vi "A33LoadArbitraryVolat.vi"(0 "VISA resource name":refnum<visa-resource-name>, 1 "ARB Number":u32=1, 3 "WFM Source":u16(ring) items=["Single file", "Split files", "Array"], 5 "Channel (1: Channel1)":u16(ring)=1 items=["Channel1"=1, "Channel2"=2], 6 "Array WFM":i16[](array[numeric]), 8 "WFM (Column) Number":i32, 9 "WFM Path":path, 11 "error in (no error)":errorcluster, 12 "WFM Length":i32, 14 "Timeout (40000 ms)":u32=40000) -> (4 "VISA resource name out":refnum<visa-resource-name>, 10 "Length of string written":i32, 15 "error out":errorcluster)   [LabVIEW 2022 SP3]
doc: "Creates and saves an arbitrary waveform in edit memory. \n\n<B>Note:</B>\n\nCreates an arbitrary waveform in edit memory and because of this, the waveform will remain stored on the instrument until deleted. If any sensitive information is contained in the arbitrary waveform, it is recommended that the waveform be deleted when finished."
uses:
  <vilib>/Utility/file.llb/Read From Spreadsheet File (I64).vi
panel:
  out "Attempts":i32
  # "Load waveform into arb\nmemory of a certain channel\nunder name 'ARB#'\nIf WFM alerady exists - use ClearArbitrary\n64M points in total per channel\nTimeout is not implemented, because this\nVI is inline-compatible, need external timeout\nincrease"
  # "No dots in the file name!"
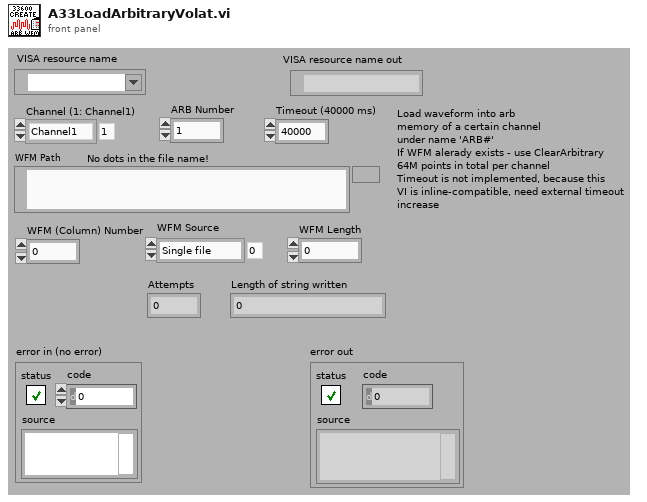
[diagram p1: front panel]
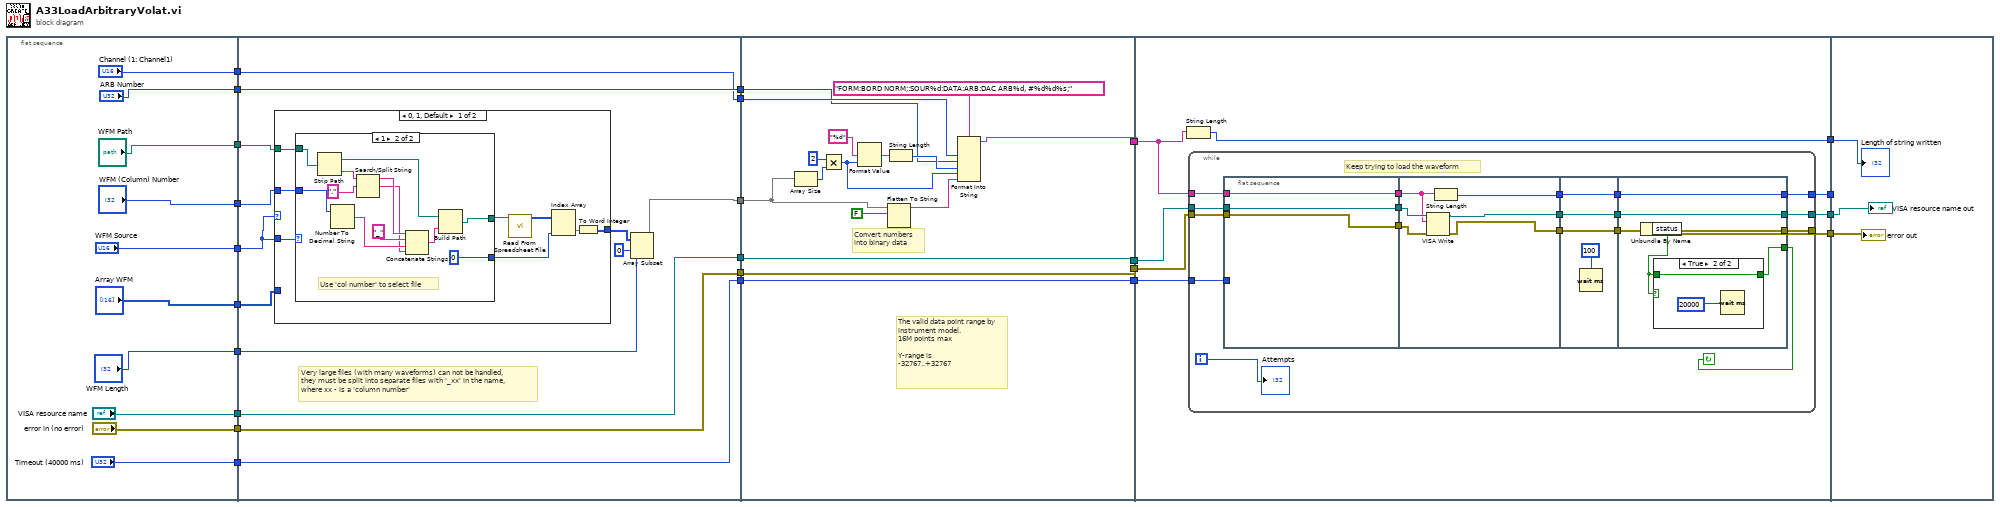
[diagram p0: block diagram]
diagram:
  n1 = flat-sequence {
    tunnel: ["Array WFM"] -> w12
    tunnel: ["WFM Source"] -> w11
    tunnel: ["ARB Number"] -> w10
    tunnel: ["Channel (1: Channel1)"] -> w9
    tunnel: ["error in (no error)"] -> w8
    tunnel: ["VISA resource name"] -> w7
    tunnel: ["Timeout (40000 ms)"] -> w6
    tunnel: ["WFM Length"] -> w5
    tunnel: ["WFM (Column) Number"] -> w4
    tunnel: ["WFM Path"] -> w3
    tunnel: [w38] -> w18
    tunnel: [w39] -> w17
    tunnel: [w40] -> w16
    tunnel: [w45] -> w15
    tunnel: [w41] -> w14
    tunnel: [w42] -> w13
    tunnel: w12 -> [w44]
    tunnel: w11 -> [w43]
    tunnel: w10 -> [w42]
    tunnel: w9 -> [w41]
    tunnel: w8 -> [w40]
    tunnel: w7 -> [w39]
    tunnel: w6 -> [w38]
    tunnel: w5 -> [w37]
    tunnel: w4 -> [w36]
    tunnel: w3 -> [w35]
    tunnel: [w86] -> w22
    tunnel: [w85] -> w21
    tunnel: [w84] -> w20
    tunnel: [w71] -> w19
    tunnel: w18 -> [w86]
    tunnel: w17 -> [w85]
    tunnel: w16 -> [w84]
    tunnel: w15 -> [w72]
    tunnel: w14 -> [w76]
    tunnel: w13 -> [w75]
    tunnel: [w91] -> w24
    tunnel: [w90] -> w23
    tunnel: w22 -> [w94]
    tunnel: w21 -> [w93]
    tunnel: w20 -> [w92]
    tunnel: w19 -> [w88]
    tunnel: [w89] -> w2
    tunnel: [w87] -> w1
    tunnel: w24 -> [w135]
    tunnel: w23 -> [w136]
    tunnel: w2 -> [_]
    tunnel: w1 -> [w134]
    frame #0 {
    }
    frame #1 {
      # "Very large files (with many waveforms) can not be handled,\nthey must be split into separate files with '_xx' in the name,\nwhere xx - is a 'column number'"
      n2 = case shown="0, 1, Default" w43 {
        tunnel: [w49 w70] -> w47
        tunnel: w35 -> [w54 _]
        tunnel: w36 -> [w53 _]
        tunnel: w43 -> [w50 _]
        tunnel: w44 -> [_ w70]
        frame 0, 1, Default {
          n3 = case shown="1" w50 {
            tunnel: w54 -> [w57 w69]
            tunnel: w53 -> [w56 w66]
            tunnel: [w57 w59] -> w52
            tunnel: [w56 0 ("x")] -> w51
            frame 0, Default {
              # "File contains multiple wfms"
            }
            frame 1 {
              # "Use 'col number' to select file"
              n4 = Strip Path(path=w69) -> (stripped path=w61:path, name=w67:string)
              n5 = Number To Decimal String(number=w66) -> (decimal integer string=w63:string)  [unwired: 1 in]
              n6 = Search/Split String(string=w67, search string/char (-)=".") -> (substring before match=w65:string, match + rest of string=w62:string)  [unwired: 1 in, 1 out]
              n7 = Concatenate Strings(w65, "_", w63, w62) -> (w60:string)
              n8 = Build Path(base path=w61, name or relative path=w60) -> (appended path=w59:path)
            }
          }
          n9 = call-poly <vilib>:"Read From Spreadsheet File.vi"("file path (dialog if empty)"=w52) -> ("all rows"=w55:i64[][])  [unwired: 6 in, 4 out]
          n10 = Index Array(array=w55, index (col)=w51) -> (element=w48:i64[])  [unwired: 1 in]
          n11 = To Word Integer(number=w48) -> (16bit integer=w49:i16[])
        }
        frame 2 {
        }
      }
      n12 = Array Subset(array=w47, index=0 ("x"), length=w37) -> (w45:i16[])
    }
    frame #2 {
      # "Convert numbers\ninto binary data"
      # "The valid data point range by instrument model. \n16M points max\n\nY-range is\n-32767..+32767"
      n13 = Array Size(array=w72) -> (size(s)=w79:i32)
      n14 = Multiply(x=2, y=w79) -> (x*y=w82:i32)
      n15 = Format Value(format string="%d", value (0)=w82) -> (output string=w80:string)  [unwired: 1 in]
      n16 = Flatten To String(anything=w72, prepend array or string size? (T)=FALSE) -> (data string=w83:string)  [unwired: 2 in, 2 out]
      n17 = String Length(string=w80) -> (length=w81:i32)
      n18 = Format Into String(format string="FORM:BORD NORM;:SOUR%d:DATA:ARB:DAC ARB%d, #%d%d%s;" ("string"), w76, w75, w81, w82, w83) -> (resulting string=w71:string)  [unwired: 2 in, 1 out]
    }
    frame #3 {
      n19 = String Length(string=w88) -> (length=w87:i32)
      n20 = while {
        tunnel: w88 -> [w109]
        tunnel: w94 -> [w108]
        tunnel: w93 -> [w107]
        tunnel: w92 -> [w106]
        tunnel: [w105] -> w91
        tunnel: [w104] -> w90
        tunnel: [w95] -> w89
        i -> [w98]
        stop <- w103 continue-if-true
        # "Keep trying to load the waveform"
        n21 = flat-sequence {
          tunnel: [w113] -> w112
          tunnel: [w114] -> w111
          tunnel: w109 -> [w115]
          tunnel: [w115] -> w110
          tunnel: w108 -> [_]
          tunnel: w107 -> [w113]
          tunnel: w106 -> [w114]
          tunnel: w112 -> [w120]
          tunnel: w111 -> [w121]
          tunnel: w110 -> [w117]
          tunnel: [w118] -> w102
          tunnel: [w119] -> w100
          tunnel: [w116] -> w96
          tunnel: w102 -> [w125]
          tunnel: [w125] -> w101
          tunnel: w100 -> [w124]
          tunnel: [w124] -> w99
          tunnel: [w122] -> w97
          tunnel: w96 -> [w122]
          tunnel: [w130] -> w104
          tunnel: [w129] -> w105
          tunnel: w101 -> [w129]
          tunnel: w99 -> [w130]
          tunnel: [w127] -> w103
          tunnel: [w126] -> w95
          tunnel: w97 -> [w126]
          frame #0 {
          }
          frame #1 {
            n22 = VISA Write(VISA resource name=w120, write buffer=w117, error in (no error)=w121) -> (VISA resource name out=w119:refnum<visa-resource-name>, error out=w118:errorcluster)  [unwired: 1 out]
            n23 = String Length(string=w117) -> (length=w116:i32)
          }
          frame #2 {
            n24 = Wait (ms)(milliseconds to wait=100 ("x")) -> ()  [unwired: 1 out]
          }
          frame #3 {
            n25 = Unbundle By Name(w129) -> ("status"=w128:bool)
            n26 = case shown="True" w128 {
              tunnel: w128 -> [w131 w132]
              tunnel: [w131 w132] -> w127
              frame False {
              }
              frame True {
                n27 = Wait (ms)(milliseconds to wait=20000 ("x")) -> ()  [unwired: 1 out]
              }
            }
          }
        }
        "Attempts" <- w98
      }
    }
    frame #4 {
      "error out" <- w135
      "VISA resource name out" <- w136
      "Length of string written" <- w134
    }
  }
